vi "Memory.Pointer.Read Bytes.vi"   [LabVIEW 2016, in "Memory.Pointer.Void.lvclass"]
uses:
  Memory.Pointer.Void.lvclass
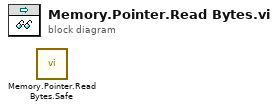
[diagram p0: block diagram]
diagram:
  n1 = call "Memory.Pointer.Read Bytes.Safe.vi"() -> ()  [unwired: 9 in, 3 out]
